vi "DPTSATKdll.vi"(8 "error in (no error)":errorcluster, 9 "kph":i32, 10 "t":dbl, 11 "icomp":i32) -> (0 "error out":errorcluster, 3 "Outputs":T1)   [LabVIEW 2015]
doc: "subroutine DPTSATKdll(icomp, t, kph, p, d, csat, dpdt, ierr, herr, herr_length)\n\nCompute the heat capacity and dP/dT along the saturation line as a function of temperature for a given component.\nSee also subroutine CSATK.\n\nINPUTS:\nicomp -- Component number in mixture (1..nc); 1 for pure fluid\nt -- Temperature [K]\nkph -- Phase flag: 1 - Liquid calculation 2 - Vapor calculation\n\nOUTPUTS:\np -- Saturated pressure [kPa]\nd -- Saturated molar density [mol/L]\ncsat -- Saturated heat capacity [J/mol-K] (same as that called from CSATK)\ndpdt -- dP/dT along the saturation line [kPa/K] (this is not dP/dT at the saturation\nline for the single phase state, but the change in saturated vapor pressure as the\nsaturation temperature changes.)\nierr -- Error flag: 0 - Successful\nherr -- Error string (character*255)\nherr_length -- length of variable herr (default: 255)"
uses:
  REFPROP.dll
panel:
  # "REFPROP-DPTSATKdll.vi"
  # "void  DPTSATKdll(int32_t *icomp, double *t, int32_t *kph, double *p, double *d, double *csat, double *dpdt, int32_t *ierr, CStr herr, int32_t herr_length);"
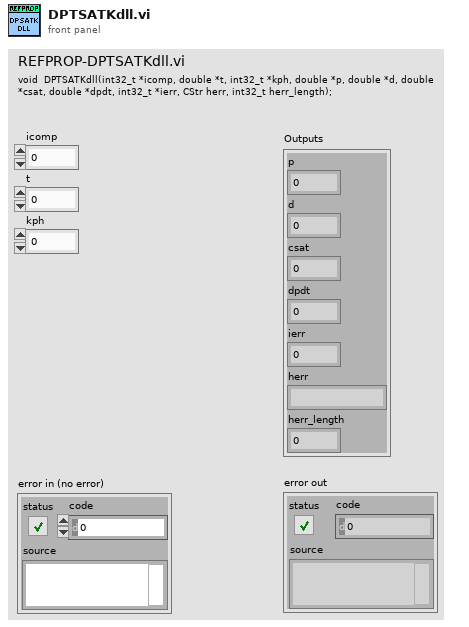
[diagram p1: front panel]
types:
  T1 = cluster{"p":dbl, "d":dbl, "csat":dbl, "dpdt":dbl, "ierr":i32, "herr":string, "herr_length":i32}
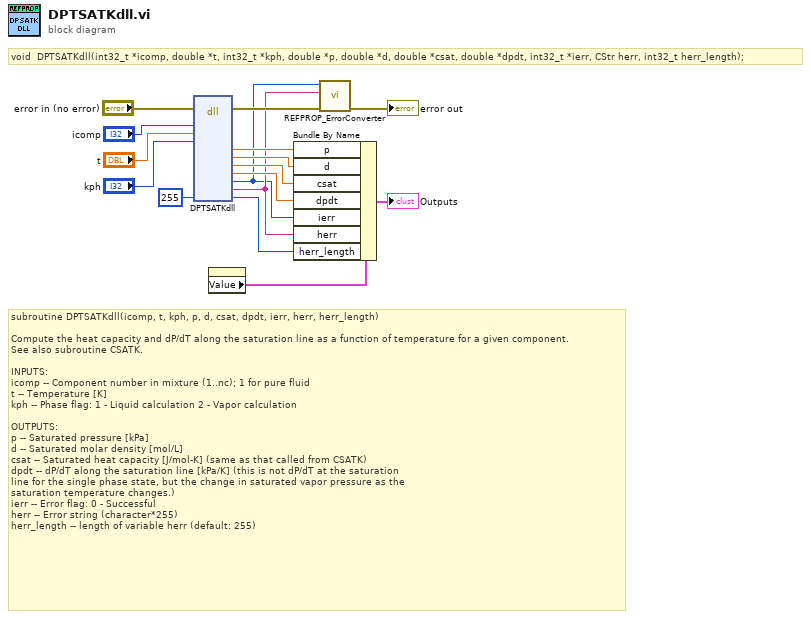
[diagram p0: block diagram]
diagram:
  # "void  DPTSATKdll(int32_t *icomp, double *t, int32_t *kph, double *p, double *d, double *csat, double *dpdt, int32_t *ierr, CStr herr, int32_t herr_length);"
  # "subroutine DPTSATKdll(icomp, t, kph, p, d, csat, dpdt, ierr, herr, herr_length)\n\nCompute the heat capacity and dP/dT along the saturation line as a function of temperature for a given component.\nSee also subroutine CSATK.\n\nINPUTS:\nicomp -- Component number in mixture (1..nc); 1 for pure fluid\nt -- Temperature [K]\nkph -- Phase flag: 1 - Liquid calculation 2 - Vapor calculation\n\nOUTPUTS:\np -- Saturated pressure [kPa]\nd -- Saturated molar density [mol/L]\ncsat -- Saturated heat capacity [J/mol-K] (same as that called from CSATK)\ndpdt -- dP/dT along the saturation line [kPa/K] (this is not dP/dT at the saturation\nline for the single phase state, but the change in saturated vapor pressure as the\nsaturation temperature changes.)\nierr -- Error flag: 0 - Successful\nherr -- Error string (character*255)\nherr_length -- length of variable herr (default: 255)"
  n1 = dll-call lib="C:/Users/lauria/Desktop/REFPROP 10 LabVIEW Wrapper BETA/REFPROP/REFPROP.*" fn="DPTSATKdll"(error in="error in (no error)", "icomp"="icomp", "t"="t", "kph"="kph", "herr_length"=255) -> (error out=w16:errorcluster, "p"=w7:dbl, "d"=w6:dbl, "csat"=w5:dbl, "dpdt"=w4:dbl, "ierr"=w1:i32, "herr"=w2:string, "herr_length"=w3:i32)  [unwired: 12 in, 1 out]
  n2 = property on="Outputs" class="Clust (strict)"() -> ("Value"=w8:T1)  [unwired: 2 in, 2 out]
  n3 = Bundle By Name(cluster=w8, "p"=w7, "d"=w6, "csat"=w5, "dpdt"=w4, "ierr"=w1, "herr"=w2, "herr_length"=w3) -> (→"Outputs":T1)
  n4 = call "REFPROP_ErrorConverter.vi"("error in (no error)"=w16, "Error Message"=w2, "Error Code"=w1) -> ("error out"=→"error out":errorcluster)  [unwired: 8 in]
